vi "_script_import_doc_txt.vi"() -> ()   [LabVIEW 2014]
uses:
  JKI State Machine++.lvlib
panel:
  out "States":string
  out "appended array":path[](array[path])
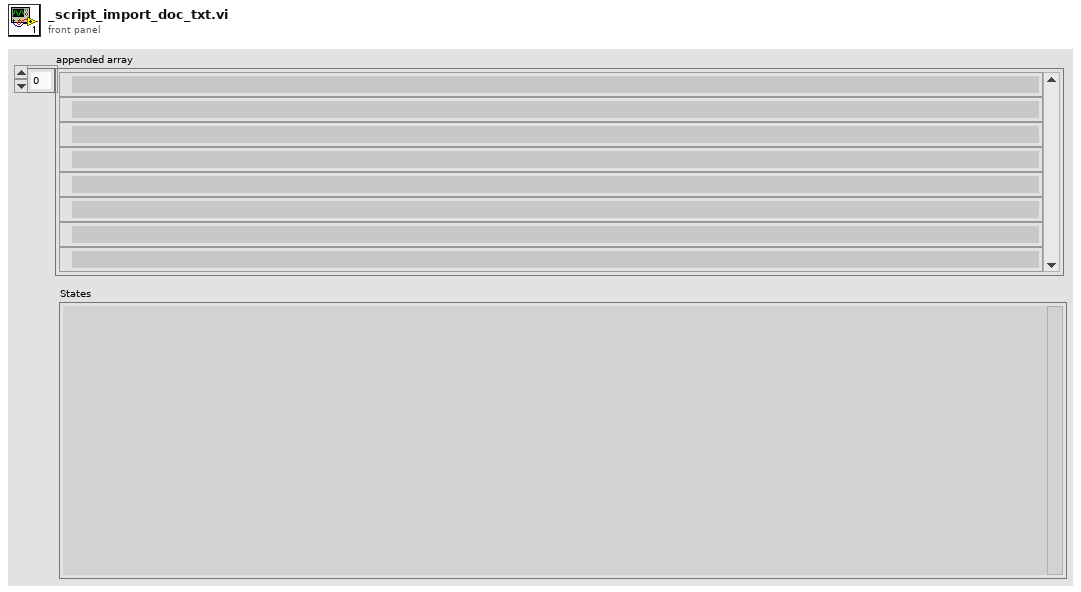
[diagram p1: front panel]
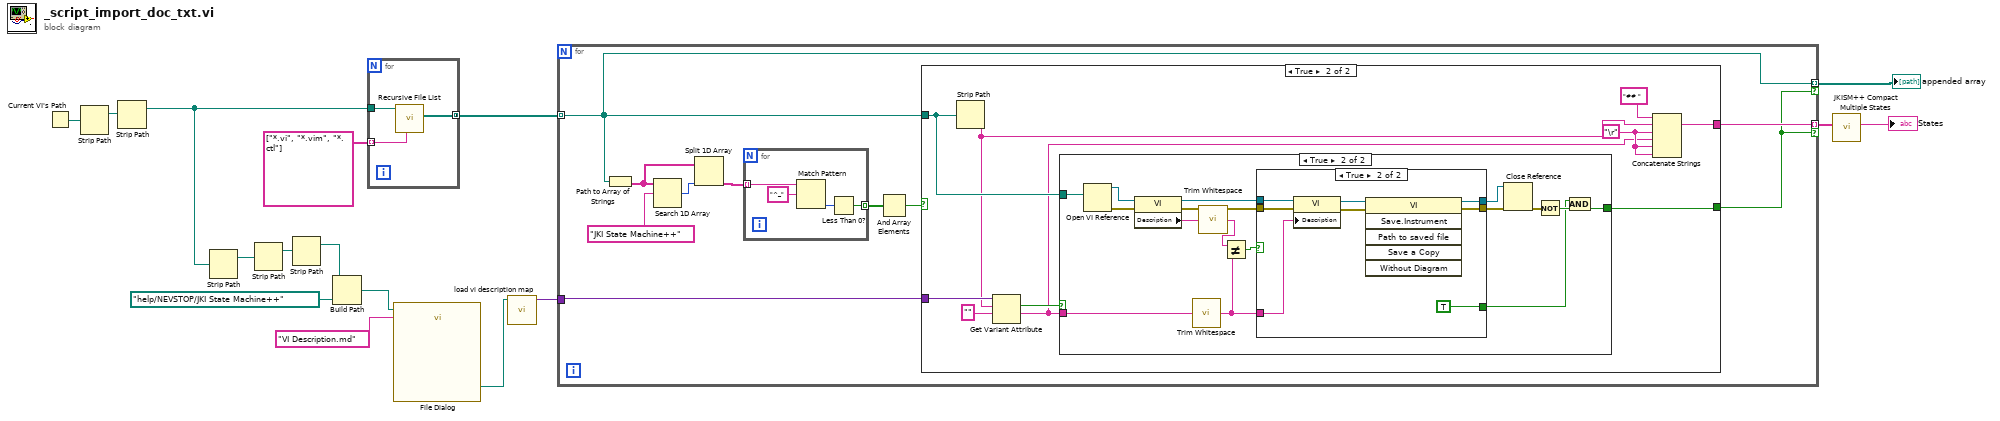
[diagram p0: block diagram]
diagram:
  n1 = Current VI's Path() -> (path=w16:path)
  n2 = Strip Path(path=w16) -> (stripped path=w15:path)  [unwired: 1 out]
  n3 = Strip Path(path=w15) -> (stripped path=w6:path)  [unwired: 1 out]
  n4 = Strip Path(path=w6) -> (stripped path=w11:path)  [unwired: 1 out]
  n5 = Strip Path(path=w11) -> (stripped path=w12:path)  [unwired: 1 out]
  n6 = Strip Path(path=w12) -> (stripped path=w9:path)  [unwired: 1 out]
  n7 = Build Path(base path=w9, name or relative path=path "help/NEVSTOP/JKI State Machine++" ("Path")) -> (appended path=w5:path)
  n8 = for {
    tunnel: w6 -> [w19]
    tunnel: string[] ["*.vi", "*.vim", "*.ctl"] -> [w18] mode=indexing
    tunnel: [w17] -> w13 mode=concatenating
    n9 = call <vilib>:"Recursive File List.vi"("pattern"=w18, "Folder Path"=w19) -> ("All Files in Dir"=w17:path[])  [unwired: 5 in, 4 out]
  }
  n10 = call "File Dialog"("start path"=w5, "default name"="VI Description.md") -> ("selected path"=w4:path)  [unwired: 10 in, 3 out]
  n11 = call "load vi description map.vi"("Path"=w4) -> ("variant"=w7:variant)  [unwired: 9 in, 1 out]
  n12 = for {
    tunnel: w13 -> [w21] mode=indexing
    tunnel: [w29] -> w8 mode=indexing if=w22
    tunnel: w7 -> [w20]
    tunnel: [w21] -> w2 mode=indexing if=w22
    n13 = Path to Array of Strings(0:w21) -> (2:w25:string[])  [unwired: 1 out]
    n14 = Search 1D Array(1D array=w25, element="JKI State Machine++") -> (index of element=w26:i32)  [unwired: 1 in]
    n15 = Split 1D Array(array=w25, index=w26) -> (second subarray=w24:string[])  [unwired: 1 out]
    n16 = for {
      tunnel: [w31] -> w28 mode=indexing
      tunnel: w24 -> [w30] mode=indexing
      n17 = Match Pattern(string=w30, regular expression="^_") -> (offset past match=w32:i32)  [unwired: 1 in, 3 out]
      n18 = Less Than 0?(x=w32) -> (x < 0?=w31:bool)
    }
    n19 = And Array Elements(Boolean array=w28) -> (logical AND=w23:bool)
    n20 = case shown="True" w23 {
      tunnel: [_ w42] -> w29
      tunnel: w21 -> [_ w39]
      tunnel: [_ w34] -> w22
      tunnel: w20 -> [_ w40]
      frame False {
      }
      frame True {
        w41 = "\r"
        n21 = Strip Path(path=w39) -> (name=w36:string)  [unwired: 1 out]
        n22 = Get Variant Attribute(Variant=w40, name=w36, default value (empty Variant)="" ("string")) -> (found=w37:bool, value=w35:string)  [unwired: 1 in, 2 out]
        n23 = case shown="True" w37 {
          tunnel: w39 -> [_ w59]
          tunnel: w35 -> [_ w58]
          tunnel: [_ w45] -> w34
          frame False {
          }
          frame True {
            n24 = Open VI Reference(vi path=w59) -> (vi reference=w52:refnum<vi>, error out=w53:errorcluster)  [unwired: 5 in]
            n25 = property class="VI"(reference=w52, error in=w53) -> (reference out=w50:refnum<vi>, error out=w51:errorcluster, "Description"=w49:string)
            n26 = call <vilib>:"Trim Whitespace.vi"("string"=w58) -> ("trimmed string"=w47:string)  [unwired: 1 in]
            n27 = call <vilib>:"Trim Whitespace.vi"("string"=w49) -> ("trimmed string"=w48:string)  [unwired: 1 in]
            n28 = Not Equal?(x=w48, y=w47) -> (x != y?=w46:bool)
            n29 = case shown="True" w46 {
              tunnel: [w61 w68] -> w57
              tunnel: [w60 w66] -> w56
              tunnel: w47 -> [_ w65]
              tunnel: w51 -> [w61 w64]
              tunnel: w50 -> [w60 w63]
              tunnel: [_ TRUE] -> w44
              frame False {
              }
              frame True {
                n30 = property class="VI"(reference=w63, error in=w64, "Description"=w65) -> (reference out=w67:refnum<vi>, error out=w69:errorcluster)
                n31 = invoke class="VI" method="Save.Instrument"(reference=w67, error in=w69) -> (reference out=w66:refnum<vi>, error out=w68:errorcluster)  [unwired: 4 in, 4 out]
              }
            }
            n32 = Close Reference(reference=w56, error in (no error)=w57) -> (error out=w55:errorcluster)
            n33 = Not(x=w55) -> (.not. x?=w54:bool)
            n34 = And(x=w44, y=w54) -> (x .and. y?=w45:bool)
          }
        }
        n35 = Concatenate Strings("## " ("string"), w36, w41, w35, w41, w41) -> (w42:string)
      }
    }
  }
  "appended array" <- w2
  n36 = call "JKISM++ Compact Multiple States.vi"("States in Lines"=w8) -> ("States"=→"States":string)  [unwired: 9 in]
